vi "SimpleContainerStartedRegAndResolve.vi"() -> ()   [LabVIEW 2024, in "Module Container.lvlib"]
uses:
  Module Container.lvlib
  ModuleCore/RQMHModule.lvclass
  ModuleCore/Show Front Panel.vi
  ModuleTemplates/NewTemplateModule/NewTemplate.lvclass
panel:
  out "error out":errorcluster
  in  "stop":bool
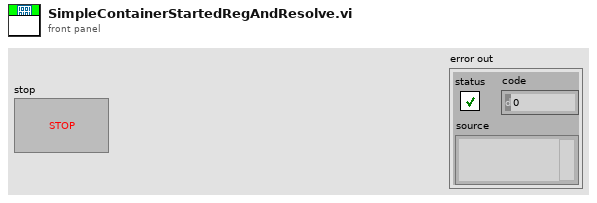
[diagram p1: front panel]
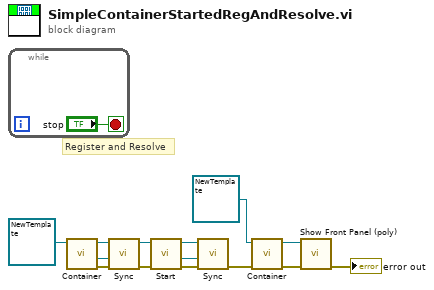
[diagram p0: block diagram]
diagram:
  # "Register and Resolve"
  n1 = while {
    stop <- "stop" stop-if-true
  }
  n2 = call "Container.vi"("Module Type"=refnum<class "NewTemplate.lvclass"> refnum ("Template")) -> ("error out"=w8:errorcluster, "Handshake (if started)"=w7:refnum<class "RQMHStartup.lvclass">, "Module Instance"=w10:refnum<class "NewTemplate.lvclass">)  [unwired: 8 in]
  n3 = call "Sync.vi"("error in (no error)"=w8, "StartupHandshake out"=w7, "JQMHCore in"=w10) -> ("error out"=w6:errorcluster, "JQMHCore out"=w13:refnum<class "NewTemplate.lvclass">)  [unwired: 7 in]
  n4 = call "Start.vi"("error in (no error)"=w6, "JQMHCore in"=w13) -> ("error out"=w14:errorcluster, "StartupHandshake out"=w11:refnum<class "RQMHStartup.lvclass">, "JQMHCore out"=w12:refnum<class "NewTemplate.lvclass">)  [unwired: 7 in]
  n5 = call "Sync.vi"("error in (no error)"=w14, "StartupHandshake out"=w11, "JQMHCore in"=w12) -> ("error out"=w9:errorcluster)  [unwired: 7 in, 1 out]
  n6 = call "Container.vi"("error in (no error)"=w9, "Module Type"=refnum<class "NewTemplate.lvclass"> refnum ("Template")) -> ("error out"=w2:errorcluster, "Module Instance"=w3:refnum<class "NewTemplate.lvclass">)  [unwired: 7 in, 1 out]
  n7 = call-poly "Show Front Panel (poly).vi"("error in (no error)"=w2, "JQMHCore in"=w3) -> ("error out"=→"error out":errorcluster)  [unwired: 8 in, 1 out]
